vi "Z_init.vi"(11 "Resource Reference":refnum<visa-resource-name>) -> (0 "error out":errorcluster, 3 "VISA Refnum out":refnum<visa-resource-name>)   [LabVIEW 2018]
doc: "Start a control session with a Hokuyo URG-04LX-UG01 device."
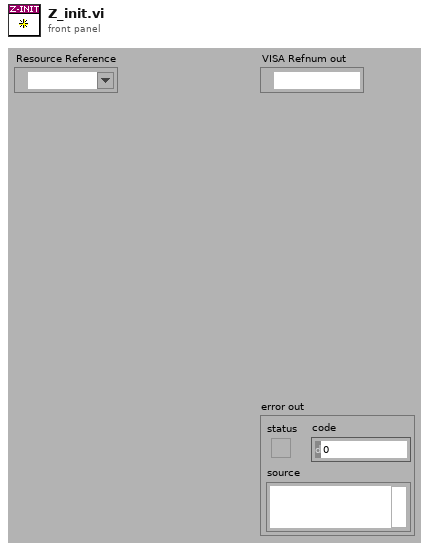
[diagram p1: front panel]
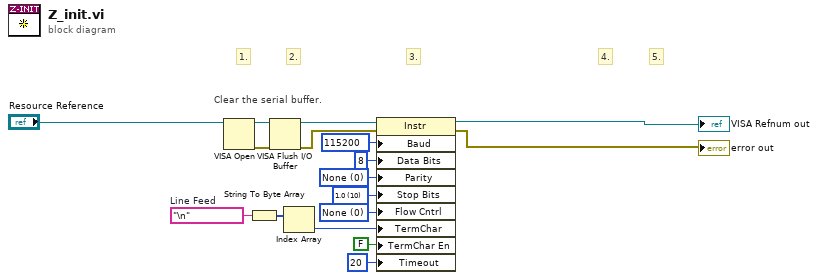
[diagram p0: block diagram]
diagram:
  w8 = "\n"  # Line Feed
  w17 = u16 0 items=["None", "XON/XOFF", "RTS/CTS", "XON/XOFF & RTS/CTS", "DTR/DSR", "XON/XOFF & DTR/DSR"] ("Serial Settings:Flow Control")
  w7 = u16 10 items=["1.0"=10, "1.5"=15, "2.0"=20] ("Serial Settings:Stop Bits")
  w6 = u16 0 items=["None", "Odd", "Even", "Mark", "Space"] ("Serial Settings:Parity")
  # "5."
  # "4."
  # "3."
  # "2."
  # "1."
  # "Clear the serial buffer."
  n1 = VISA Open(VISA resource name="Resource Reference") -> (VISA resource name=w12:refnum<visa-resource-name>, error out=w13:errorcluster)  [unwired: 4 in]
  n2 = String To Byte Array(string=w8) -> (unsigned byte array=w9:u8[])
  n3 = VISA Flush I/O Buffer(VISA resource name=w12, error in (no error)=w13) -> (VISA resource name out=w15:refnum<visa-resource-name>, error out=w14:errorcluster)  [unwired: 1 in]
  n4 = Index Array(array=w9) -> (element=w10:u8)  [unwired: 1 in]
  n5 = property class="Instr"(reference=w15, error in=w14, "Baud"=u32 115200 ("Serial Settings:Baud Rate"), "Data Bits"=u16 8 ("Serial Settings:Data Bits"), "Parity"=w6, "Stop Bits"=w7, "Flow Cntrl"=w17, "TermChar"=w10, "TermChar En"=FALSE ("Message Based Settings:Termination Character Enable"), "Timeout"=u32 20 ("General Settings:Timeout Value")) -> (reference out=→"VISA Refnum out":refnum<visa-resource-name>, error out=→"error out":errorcluster)
